vi "TDMs Ref.vi"(7 "Ini?":bool, 8 "error in (no error)":errorcluster caption="错误输入（无错误）", 11 "tdms file out":refnum<k34>) -> (0 "error out":errorcluster caption="错误输出", 3 "tdms file out":refnum<k34>)   [LabVIEW 2012]
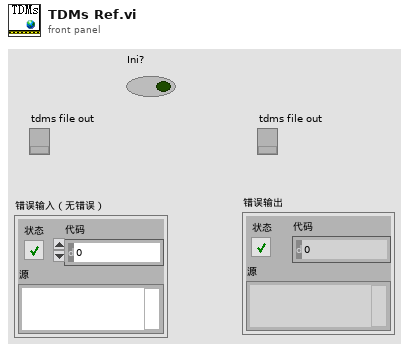
[diagram p1: front panel]
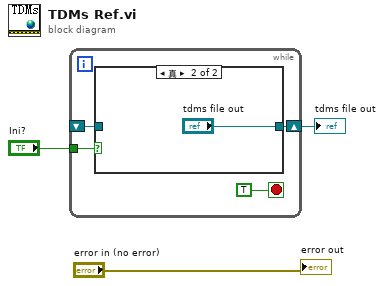
[diagram p0: block diagram]
diagram:
  n1 = while {
    tunnel: "Ini?" -> [w6]
    shift-right: [w5] -> w2
    shift-left: _ -> [w4]
    stop <- TRUE stop-if-true
    n2 = case shown="真" w6 {
      tunnel: [w8 "tdms file out"] -> w5
      tunnel: w4 -> [w8 _]
      frame False {
      }
      frame True {
      }
    }
  }
  "tdms file out" <- w2
  "error out" <- "error in (no error)"
